vi "DAQAssist-2.vi"(0 "Calibration Array":dbl[](array[numeric]), 1 "number of samples":i32, 2 "rate":dbl, 3 "error in":errorcluster, 4 "stopped":bool) -> (5 "Dynamic Data Type":dynamicdata(waveform), 6 "error out":errorcluster)   [LabVIEW 2012]
uses:
  <vilib>/DAQmx/read.llb/DAQmx Read (Analog 1D Wfm NChan NSamp).vi
  <vilib>/DAQmx/create/channels.llb/DAQmx Create Channel (TEDS-AI-Voltage-Basic).vi
  <vilib>/DAQmx/create/channels.llb/DAQmx Create Channel (AI-Voltage-Basic).vi
  <vilib>/DAQmx/create/channels.llb/DAQmx Create Channel (TEDS-AI-Acceleration-Accelerometer).vi
  <vilib>/DAQmx/create/channels.llb/DAQmx Create Channel (AI-Acceleration-Accelerometer).vi
  <vilib>/DAQmx/configure/timing.llb/DAQmx Timing (Sample Clock).vi
  <vilib>/DAQmx/miscellaneous.llb/DAQmx Fill In Error Info.vi
  <resource>/objmgr/daqmx.rc
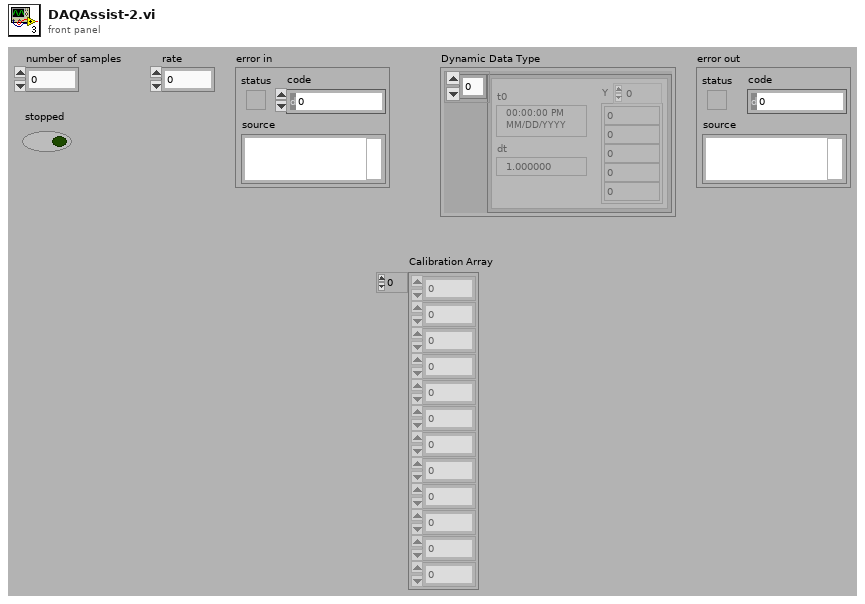
[diagram p1: front panel]
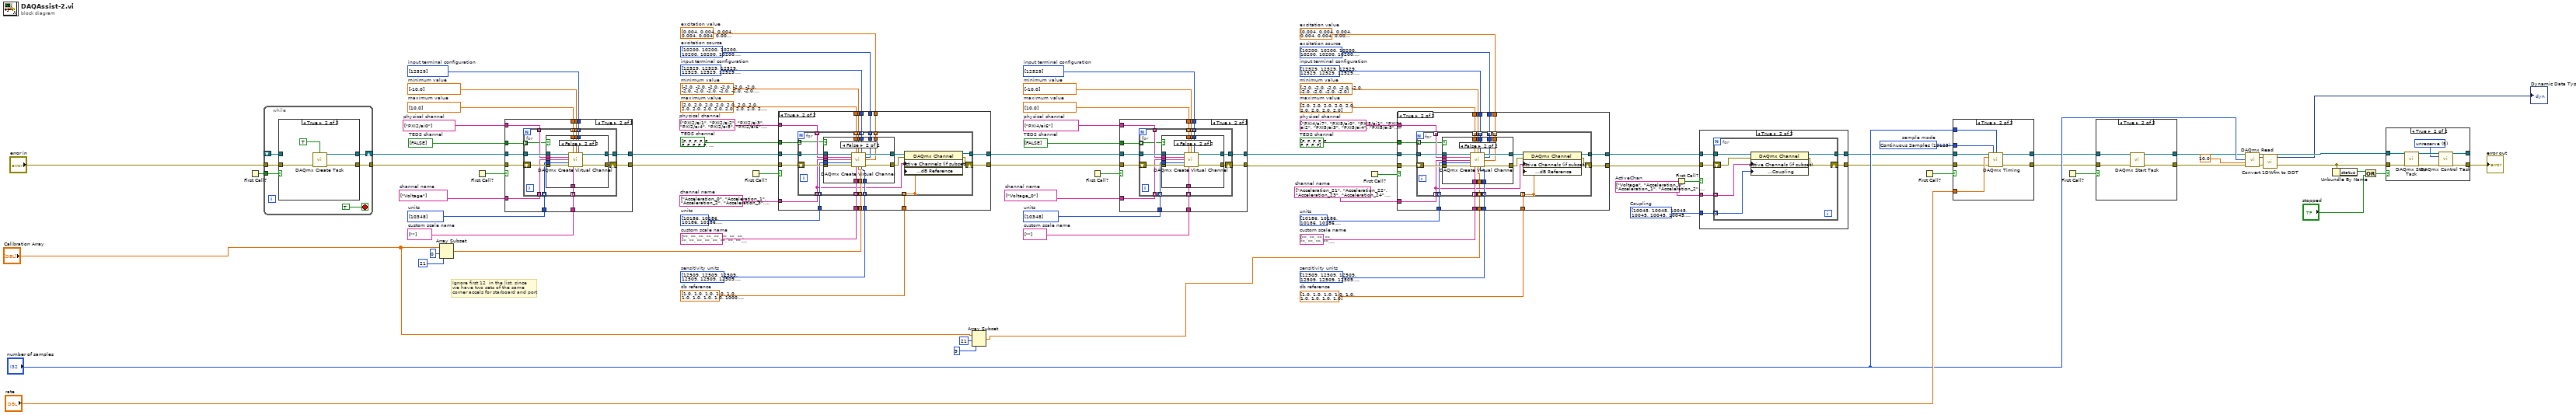
[diagram p0: block diagram]
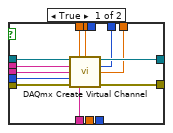
[diagram p3: hidden frame]
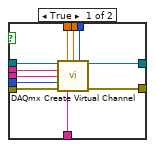
[diagram p5: hidden frame]
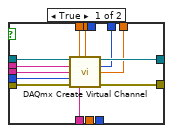
[diagram p11: hidden frame]
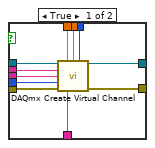
[diagram p13: hidden frame]
diagram:
  w9 = string[] ["Acceleration_21", "Acceleration_22", "Acceleration_23", "Acceleration_24", "Acceleration_25", "Acceleration_26", "Acceleration_27", "Acceleration_28", "Acceleration_29"]  # channel name
  w10 = string[] ["Voltage_0"]  # channel name
  w11 = string[] ["Acceleration_0", "Acceleration_1", "Acceleration_2", "Acceleration_3", "Acceleration_4", "Acceleration_5", "Acceleration_6", "Acceleration_7", "Acceleration_8", "Acceleration_9", "Acceleration_10", "Acceleration_11", "Acceleration_12", "Acceleration_13", "Acceleration_14", "Acceleration_15", "Acceleration_16", "Acceleration_17", "Acceleration_18", "Acceleration_19", "Acceleration_20"]  # channel name
  w12 = string[] ["PXI2/ai1", "PXI2/ai2", "PXI2/ai3", "PXI2/ai4", "PXI2/ai5", "PXI2/ai6", "PXI2/ai7", "PXI3/ai0", "PXI3/ai1", "PXI3/ai2", "PXI3/ai3", "PXI3/ai4", "PXI3/ai5", "PXI3/ai6", "PXI3/ai7", "PXI4/ai0", "PXI4/ai1", "PXI4/ai2", "PXI4/ai3", "PXI4/ai4", "PXI4/ai5"]  # physical channel
  w13 = string[] ["Voltage"]  # channel name
  w14 = string[] ["PXI2/ai0"]  # physical channel
  w15 = i32[] [10045, 10045, 10045, 10045, 10045, 10045, 10045, 10045, 10045, 10045, 10045, 10045, 10045, 10045, 10045, 10045, 10045, 10045, 10045, 10045, 10045, 10045, 10045, 10045, 10045, 10045, 10045, 10045, 10045, 10045, 10045, 10045] items=["AC"=10045, "DC"=10050, "GND"=10066]  # Coupling
  w16 = string[] ["Voltage", "Acceleration_0", "Acceleration_1", "Acceleration_2", "Acceleration_3", "Acceleration_4", "Acceleration_5", "Acceleration_6", "Acceleration_7", "Acceleration_8", "Acceleration_9", "Acceleration_10", "Acceleration_11", "Acceleration_12", "Acceleration_13", "Acceleration_14", "Acceleration_15", "Acceleration_16", "Acceleration_17", "Acceleration_18", "Acceleration_19", "Acceleration_20", "Voltage_0", "Acceleration_21", "Acceleration_22", "Acceleration_23", "Acceleration_24", "Acceleration_25", "Acceleration_26", "Acceleration_27", "Acceleration_28", "Acceleration_29"]  # ActiveChan
  w32 = dbl[] [1.0, 1.0, 1.0, 1.0, 1.0, 1.0, 1.0, 1.0, 1.0]  # db reference
  w31 = bool[] [FALSE, FALSE, FALSE, FALSE, FALSE, FALSE, FALSE, FALSE, FALSE]  # TEDS channel
  w30 = i32[] [12529, 12529, 12529, 12529, 12529, 12529, 12529, 12529, 12529] items=["default"=-1, "RSE"=10083, "NRSE"=10078, "Differential"=10106, "Pseudodifferential"=12529]  # input terminal configuration
  w28 = i32[] [10200, 10200, 10200, 10200, 10200, 10200, 10200, 10200, 10200] items=["Internal"=10200, "External"=10167, "None"=10230]  # excitation source
  w29 = i32[] [12509, 12509, 12509, 12509, 12509, 12509, 12509, 12509, 12509] items=["mVolts/g"=12509, "Volts/g"=12510]  # sensitivity units
  w27 = dbl[] [0.004, 0.004, 0.004, 0.004, 0.004, 0.004, 0.004, 0.004, 0.004]  # excitation value
  w26 = string[] ["", "", "", "", "", "", "", "", ""]  # custom scale name
  w25 = i32[] [10186, 10186, 10186, 10186, 10186, 10186, 10186, 10186, 10186] items=["g"=10186, "m/s^2"=12470, "From Custom Scale"=10065]  # units
  w24 = string[] ["PXI4/ai7", "PXI5/ai0", "PXI5/ai1", "PXI5/ai2", "PXI5/ai3", "PXI5/ai4", "PXI5/ai5", "PXI5/ai6", "PXI5/ai7"]  # physical channel
  w23 = dbl[] [2.0, 2.0, 2.0, 2.0, 2.0, 2.0, 2.0, 2.0, 2.0]  # maximum value
  w22 = dbl[] [-2.0, -2.0, -2.0, -2.0, -2.0, -2.0, -2.0, -2.0, -2.0]  # minimum value
  w42 = bool[] [FALSE]  # TEDS channel
  w41 = string[] [""]  # custom scale name
  w40 = i32[] [10348] items=["Volts"=10348, "From TEDS"=12516, "From Custom Scale"=10065]  # units
  w39 = string[] ["PXI4/ai6"]  # physical channel
  w38 = dbl[] [10.0]  # maximum value
  w37 = dbl[] [-10.0]  # minimum value
  w36 = i32[] [12529] items=["default"=-1, "RSE"=10083, "NRSE"=10078, "Differential"=10106, "Pseudodifferential"=12529]  # input terminal configuration
  w72 = 10123 items=["Finite Samples"=10178, "Continuous Samples"=10123, "Hardware Timed Single Point"=12522]  # sample mode
  w66 = dbl[] [1.0, 1.0, 1.0, 1.0, 1.0, 1.0, 1.0, 1.0, 1.0, 1000.0, 1000.0, 1000.0, 1000.0, 1000.0, 1000.0, 1000.0, 1000.0, 1000.0, 1000.0, 1000.0, 1.0]  # db reference
  w65 = bool[] [FALSE, FALSE, FALSE, FALSE, FALSE, FALSE, FALSE, FALSE, FALSE, FALSE, FALSE, FALSE, FALSE, FALSE, FALSE, FALSE, FALSE, FALSE, FALSE, FALSE, FALSE]  # TEDS channel
  w64 = i32[] [12529, 12529, 12529, 12529, 12529, 12529, 12529, 12529, 12529, 12529, 12529, 12529, 12529, 12529, 12529, 12529, 12529, 12529, 12529, 12529, 12529] items=["default"=-1, "RSE"=10083, "NRSE"=10078, "Differential"=10106, "Pseudodifferential"=12529]  # input terminal configuration
  w62 = i32[] [10200, 10200, 10200, 10200, 10200, 10200, 10200, 10200, 10200, 10200, 10200, 10200, 10200, 10200, 10200, 10200, 10200, 10200, 10200, 10200, 10200] items=["Internal"=10200, "External"=10167, "None"=10230]  # excitation source
  w63 = i32[] [12509, 12509, 12509, 12509, 12509, 12509, 12509, 12509, 12509, 12509, 12509, 12509, 12509, 12509, 12509, 12509, 12509, 12509, 12509, 12509, 12509] items=["mVolts/g"=12509, "Volts/g"=12510]  # sensitivity units
  w61 = dbl[] [0.004, 0.004, 0.004, 0.004, 0.004, 0.004, 0.004, 0.004, 0.004, 0.004, 0.004, 0.004, 0.004, 0.004, 0.004, 0.004, 0.004, 0.004, 0.004, 0.004, 0.004]  # excitation value
  w60 = string[] ["", "", "", "", "", "", "", "", "", "", "", "", "", "", "", "", "", "", "", "", ""]  # custom scale name
  w59 = i32[] [10186, 10186, 10186, 10186, 10186, 10186, 10186, 10186, 10186, 10186, 10186, 10186, 10186, 10186, 10186, 10186, 10186, 10186, 10186, 10186, 10186] items=["g"=10186, "m/s^2"=12470, "From Custom Scale"=10065]  # units
  w58 = dbl[] [2.0, 2.0, 2.0, 2.0, 2.0, 2.0, 2.0, 2.0, 2.0, 2.0, 2.0, 2.0, 2.0, 2.0, 2.0, 2.0, 2.0, 2.0, 2.0, 2.0, 2.0]  # maximum value
  w57 = dbl[] [-2.0, -2.0, -2.0, -2.0, -2.0, -2.0, -2.0, -2.0, -2.0, -2.0, -2.0, -2.0, -2.0, -2.0, -2.0, -2.0, -2.0, -2.0, -2.0, -2.0, -2.0]  # minimum value
  w54 = bool[] [FALSE]  # TEDS channel
  w53 = string[] [""]  # custom scale name
  w52 = i32[] [10348] items=["Volts"=10348, "From TEDS"=12516, "From Custom Scale"=10065]  # units
  w51 = dbl[] [10.0]  # maximum value
  w50 = dbl[] [-10.0]  # minimum value
  w49 = i32[] [12529] items=["default"=-1, "RSE"=10083, "NRSE"=10078, "Differential"=10106, "Pseudodifferential"=12529]  # input terminal configuration
  # "Ignore first 12  in the list, since \nwe have two sets of the same \ncorner accels for starboard and port"
  n1 = First Call?() -> (First Call?: T/F=w43:bool)
  n2 = while {
    shift-right: [w91] -> w47
    shift-left: _ -> [w90]
    tunnel: w43 -> [w92]
    tunnel: [w89] -> w44
    tunnel: "error in" -> [w88]
    stop <- TRUE stop-if-true
    n3 = case shown="True" w92 {
      tunnel: [w94 w98] -> w91
      tunnel: w90 -> [w94 _]
      tunnel: [w93 w97] -> w89
      tunnel: w88 -> [w93 w95]
      frame False {
      }
      frame True {
        n4 = call <vilib>:"DAQmx Create Task.vi"("auto cleanup"=TRUE, "error in"=w95) -> ("task out"=w98:refnum<k21>, "error out"=w97:errorcluster)  [unwired: 12 in]
      }
    }
  }
  n5 = Array Subset(array="Calibration Array", index=0, length=21) -> (w6:dbl[])
  n6 = First Call?() -> (First Call?: T/F=w46:bool)
  n7 = case shown="True" w46 {
    tunnel: [w100 w110] -> w56
    tunnel: w47 -> [w100 w112]
    tunnel: [w99 w109] -> w48
    tunnel: w44 -> [w99 w111]
    tunnel: w49 -> [_ w108]
    tunnel: w50 -> [_ w107]
    tunnel: w51 -> [_ w106]
    tunnel: w14 -> [_ w105]
    tunnel: w13 -> [_ w104]
    tunnel: w52 -> [_ w103]
    tunnel: w53 -> [_ w102]
    tunnel: w54 -> [_ w101]
    frame False {
    }
    frame True {
      n8 = for {
        tunnel: w112 -> [w124]
        tunnel: [w122] -> w110
        tunnel: w108 -> [w120] mode=indexing
        tunnel: w107 -> [w119] mode=indexing
        tunnel: w106 -> [w118] mode=indexing
        tunnel: w105 -> [w117] mode=indexing
        tunnel: w104 -> [w116] mode=indexing
        tunnel: w103 -> [w115] mode=indexing
        tunnel: w102 -> [w114] mode=indexing
        shift-right: [w121] -> w109
        shift-left: w111 -> [w123]
        tunnel: w101 -> [w113] mode=indexing
        n9 = case shown="False" w113 {
          tunnel: w124 -> [w135 w146]
          tunnel: w123 -> [w134 w145]
          tunnel: [w133 w144] -> w122
          tunnel: [w132 w143] -> w121
          tunnel: w120 -> [w131 w142]
          tunnel: w119 -> [w130 w141]
          tunnel: w118 -> [w129 w140]
          tunnel: w117 -> [w128 w139]
          tunnel: w116 -> [w127 w138]
          tunnel: w115 -> [w126 w137]
          tunnel: w114 -> [w125 w136]
          frame True {
            n10 = call-poly <vilib>:"DAQmx Create Virtual Channel.vi"("task in"=w135, "maximum value"=w129, "minimum value"=w130, "input terminal configuration"=w131, "physical channels"=w128, "name to assign"=w127, "units"=w126, "error in"=w134, "custom scale name"=w125) -> ("task out"=w133:refnum<k21>, "error out"=w132:errorcluster)  [unwired: 5 in]
          }
          frame False {
            n11 = call-poly <vilib>:"DAQmx Create Virtual Channel.vi"("task in"=w146, "maximum value"=w140, "minimum value"=w141, "input terminal configuration"=w142, "physical channels"=w139, "name to assign"=w138, "units"=w137, "error in"=w145, "custom scale name"=w136) -> ("task out"=w144:refnum<k21>, "error out"=w143:errorcluster)  [unwired: 5 in]
          }
        }
      }
    }
  }
  n12 = First Call?() -> (First Call?: T/F=w55:bool)
  n13 = case shown="True" w55 {
    tunnel: [w148 w163] -> w34
    tunnel: w56 -> [w148 w165]
    tunnel: [w147 w162] -> w33
    tunnel: w48 -> [w147 w164]
    tunnel: w57 -> [_ w161]
    tunnel: w58 -> [_ w160]
    tunnel: w12 -> [_ w159]
    tunnel: w11 -> [_ w158]
    tunnel: w59 -> [_ w157]
    tunnel: w60 -> [_ w156]
    tunnel: w61 -> [_ w155]
    tunnel: w62 -> [_ w154]
    tunnel: w6 -> [_ w153]
    tunnel: w63 -> [_ w152]
    tunnel: w64 -> [_ w151]
    tunnel: w65 -> [_ w150]
    tunnel: w66 -> [_ w149]
    frame False {
    }
    frame True {
      n14 = for {
        tunnel: w165 -> [w184]
        tunnel: [w170] -> w163
        tunnel: w161 -> [w182] mode=indexing
        tunnel: w160 -> [w181] mode=indexing
        tunnel: w159 -> [w180] mode=indexing
        tunnel: w158 -> [w166] mode=indexing
        tunnel: w157 -> [w179] mode=indexing
        tunnel: w156 -> [w178] mode=indexing
        shift-right: [w169] -> w162
        shift-left: w164 -> [w183]
        tunnel: w155 -> [w177] mode=indexing
        tunnel: w154 -> [w176] mode=indexing
        tunnel: w153 -> [w175] mode=indexing
        tunnel: w152 -> [w174] mode=indexing
        tunnel: w151 -> [w173] mode=indexing
        tunnel: w150 -> [w172] mode=indexing
        tunnel: [w167] -> _ mode=indexing
        tunnel: w149 -> [w167] mode=indexing
        n15 = case shown="False" w172 {
          tunnel: w184 -> [w196 w211]
          tunnel: w183 -> [w195 w210]
          tunnel: [w194 w209] -> w171
          tunnel: [w193 w208] -> w168
          tunnel: w182 -> [w192 w207]
          tunnel: w181 -> [w191 w206]
          tunnel: w180 -> [w190 w205]
          tunnel: w166 -> [w189 w204]
          tunnel: w179 -> [w188 w203]
          tunnel: w178 -> [w187 w202]
          tunnel: w177 -> [w186 w201]
          tunnel: w176 -> [w185 w200]
          tunnel: w175 -> [_ w199]
          tunnel: w174 -> [_ w198]
          tunnel: w173 -> [_ w197]
          frame True {
            n16 = call-poly <vilib>:"DAQmx Create Virtual Channel.vi"("task in"=w196, "maximum value"=w191, "minimum value"=w192, "physical channels"=w190, "current excitation source"=w185, "name to assign"=w189, "current excitation value"=w186, "units"=w188, "error in"=w195, "custom scale name"=w187) -> ("task out"=w194:refnum<k21>, "error out"=w193:errorcluster)  [unwired: 4 in]
          }
          frame False {
            n17 = call-poly <vilib>:"DAQmx Create Virtual Channel.vi"("task in"=w211, "maximum value"=w206, "minimum value"=w207, "input terminal configuration"=w197, "physical channels"=w205, "current excitation source"=w200, "name to assign"=w204, "current excitation value"=w201, "units"=w203, "error in"=w210, "custom scale name"=w202, "sensitivity"=w199, "sensitivity units"=w198) -> ("task out"=w209:refnum<k21>, "error out"=w208:errorcluster)  [unwired: 1 in]
          }
        }
        n18 = property class="DAQmx Channel"(reference=w171, error in=w168, "Active Channels (if subset)"=w166, "Analog Input:Acceleration:dB Reference"=w167) -> (reference out=w170:refnum<k21>, error out=w169:errorcluster)
      }
    }
  }
  n19 = Array Subset(array="Calibration Array", index=21, length=9) -> (w2:dbl[])
  n20 = First Call?() -> (First Call?: T/F=w35:bool)
  n21 = case shown="True" w35 {
    tunnel: [w213 w223] -> w20
    tunnel: w34 -> [w213 w225]
    tunnel: [w212 w222] -> w19
    tunnel: w33 -> [w212 w224]
    tunnel: w36 -> [_ w221]
    tunnel: w37 -> [_ w220]
    tunnel: w38 -> [_ w219]
    tunnel: w39 -> [_ w218]
    tunnel: w10 -> [_ w217]
    tunnel: w40 -> [_ w216]
    tunnel: w41 -> [_ w215]
    tunnel: w42 -> [_ w214]
    frame False {
    }
    frame True {
      n22 = for {
        tunnel: w225 -> [w237]
        tunnel: [w235] -> w223
        tunnel: w221 -> [w233] mode=indexing
        tunnel: w220 -> [w232] mode=indexing
        tunnel: w219 -> [w231] mode=indexing
        tunnel: w218 -> [w230] mode=indexing
        tunnel: w217 -> [w229] mode=indexing
        tunnel: w216 -> [w228] mode=indexing
        tunnel: w215 -> [w227] mode=indexing
        shift-right: [w234] -> w222
        shift-left: w224 -> [w236]
        tunnel: w214 -> [w226] mode=indexing
        n23 = case shown="False" w226 {
          tunnel: w237 -> [w248 w259]
          tunnel: w236 -> [w247 w258]
          tunnel: [w246 w257] -> w235
          tunnel: [w245 w256] -> w234
          tunnel: w233 -> [w244 w255]
          tunnel: w232 -> [w243 w254]
          tunnel: w231 -> [w242 w253]
          tunnel: w230 -> [w241 w252]
          tunnel: w229 -> [w240 w251]
          tunnel: w228 -> [w239 w250]
          tunnel: w227 -> [w238 w249]
          frame True {
            n24 = call-poly <vilib>:"DAQmx Create Virtual Channel.vi"("task in"=w248, "maximum value"=w242, "minimum value"=w243, "input terminal configuration"=w244, "physical channels"=w241, "name to assign"=w240, "units"=w239, "error in"=w247, "custom scale name"=w238) -> ("task out"=w246:refnum<k21>, "error out"=w245:errorcluster)  [unwired: 5 in]
          }
          frame False {
            n25 = call-poly <vilib>:"DAQmx Create Virtual Channel.vi"("task in"=w259, "maximum value"=w253, "minimum value"=w254, "input terminal configuration"=w255, "physical channels"=w252, "name to assign"=w251, "units"=w250, "error in"=w258, "custom scale name"=w249) -> ("task out"=w257:refnum<k21>, "error out"=w256:errorcluster)  [unwired: 5 in]
          }
        }
      }
    }
  }
  n26 = First Call?() -> (First Call?: T/F=w21:bool)
  n27 = case shown="True" w21 {
    tunnel: [w261 w276] -> w18
    tunnel: w20 -> [w261 w278]
    tunnel: [w260 w275] -> w17
    tunnel: w19 -> [w260 w277]
    tunnel: w22 -> [_ w274]
    tunnel: w23 -> [_ w273]
    tunnel: w24 -> [_ w272]
    tunnel: w9 -> [_ w271]
    tunnel: w25 -> [_ w270]
    tunnel: w26 -> [_ w269]
    tunnel: w27 -> [_ w268]
    tunnel: w28 -> [_ w267]
    tunnel: w29 -> [_ w266]
    tunnel: w30 -> [_ w265]
    tunnel: w31 -> [_ w264]
    tunnel: w32 -> [_ w263]
    tunnel: w2 -> [_ w262]
    frame False {
    }
    frame True {
      n28 = for {
        tunnel: w278 -> [w297]
        tunnel: [w284] -> w276
        tunnel: w274 -> [w295] mode=indexing
        tunnel: w273 -> [w294] mode=indexing
        tunnel: w272 -> [w293] mode=indexing
        tunnel: w271 -> [w280] mode=indexing
        tunnel: w270 -> [w292] mode=indexing
        tunnel: w269 -> [w291] mode=indexing
        shift-right: [w283] -> w275
        shift-left: w277 -> [w296]
        tunnel: w268 -> [w290] mode=indexing
        tunnel: w267 -> [w289] mode=indexing
        tunnel: w266 -> [w288] mode=indexing
        tunnel: w265 -> [w287] mode=indexing
        tunnel: w264 -> [w286] mode=indexing
        tunnel: [w281] -> _ mode=indexing
        tunnel: w263 -> [w281] mode=indexing
        tunnel: w262 -> [w279] mode=indexing
        n29 = case shown="False" w286 {
          tunnel: w297 -> [w309 w324]
          tunnel: w296 -> [w308 w323]
          tunnel: [w307 w322] -> w285
          tunnel: [w306 w321] -> w282
          tunnel: w295 -> [w305 w320]
          tunnel: w294 -> [w304 w319]
          tunnel: w293 -> [w303 w318]
          tunnel: w280 -> [w302 w317]
          tunnel: w292 -> [w301 w316]
          tunnel: w291 -> [w300 w315]
          tunnel: w290 -> [w299 w314]
          tunnel: w289 -> [w298 w313]
          tunnel: w288 -> [_ w312]
          tunnel: w287 -> [_ w311]
          tunnel: w279 -> [_ w310]
          frame True {
            n30 = call-poly <vilib>:"DAQmx Create Virtual Channel.vi"("task in"=w309, "maximum value"=w304, "minimum value"=w305, "physical channels"=w303, "current excitation source"=w298, "name to assign"=w302, "current excitation value"=w299, "units"=w301, "error in"=w308, "custom scale name"=w300) -> ("task out"=w307:refnum<k21>, "error out"=w306:errorcluster)  [unwired: 4 in]
          }
          frame False {
            n31 = call-poly <vilib>:"DAQmx Create Virtual Channel.vi"("task in"=w324, "maximum value"=w319, "minimum value"=w320, "input terminal configuration"=w311, "physical channels"=w318, "current excitation source"=w313, "name to assign"=w317, "current excitation value"=w314, "units"=w316, "error in"=w323, "custom scale name"=w315, "sensitivity"=w310, "sensitivity units"=w312) -> ("task out"=w322:refnum<k21>, "error out"=w321:errorcluster)  [unwired: 1 in]
          }
        }
        n32 = property class="DAQmx Channel"(reference=w285, error in=w282, "Active Channels (if subset)"=w280, "Analog Input:Acceleration:dB Reference"=w281) -> (reference out=w284:refnum<k21>, error out=w283:errorcluster)
      }
    }
  }
  n33 = First Call?() -> (First Call?: T/F=w68:bool)
  n34 = case shown="True" w68 {
    tunnel: w18 -> [w326 w332]
    tunnel: w17 -> [w325 w331]
    tunnel: [w326 w330] -> w70
    tunnel: [w325 w329] -> w67
    tunnel: w16 -> [_ w328]
    tunnel: w15 -> [_ w327]
    frame False {
    }
    frame True {
      n35 = for {
        tunnel: w332 -> [w338]
        tunnel: [w336] -> w330
        tunnel: w328 -> [w334] mode=indexing
        shift-right: [w335] -> w329
        shift-left: w331 -> [w337]
        tunnel: w327 -> [w333] mode=indexing
        n36 = property class="DAQmx Channel"(reference=w338, error in=w337, "Active Channels (if subset)"=w334, "Analog Input:General Properties:Input Configuration:Coupling"=w333) -> (reference out=w336:refnum<k21>, error out=w335:errorcluster)
      }
    }
  }
  n37 = First Call?() -> (First Call?: T/F=w69:bool)
  n38 = case shown="True" w69 {
    tunnel: [w340 w342] -> w74
    tunnel: w70 -> [w340 w345]
    tunnel: [w339 w341] -> w71
    tunnel: w67 -> [w339 w343]
    tunnel: "number of samples" -> [_ w347]
    tunnel: w72 -> [_ w346]
    tunnel: "rate" -> [_ w344]
    frame False {
    }
    frame True {
      n39 = call-poly <vilib>:"DAQmx Timing.vi"("task/channels in"=w345, "sample mode"=w346, "samples per channel"=w347, "rate"=w344, "error in"=w343) -> ("task out"=w342:refnum<k21>, "error out"=w341:errorcluster)  [unwired: 9 in]
    }
  }
  n40 = First Call?() -> (First Call?: T/F=w73:bool)
  n41 = case shown="True" w73 {
    tunnel: [w349 w352] -> w77
    tunnel: w74 -> [w349 w353]
    tunnel: [w348 w350] -> w75
    tunnel: w71 -> [w348 w351]
    frame False {
    }
    frame True {
      n42 = call <vilib>:"DAQmx Start Task.vi"("task/channels in"=w353, "error in"=w351) -> ("task out"=w352:refnum<k21>, "error out"=w350:errorcluster)  [unwired: 12 in]
    }
  }
  n43 = call-poly <vilib>:"DAQmx Read.vi"("task/channels in"=w77, "number of samples per channel"="number of samples", "timeout"=10.0, "error in"=w75) -> ("task out"=w81:refnum<k21>, "data"=w79:waveform(dbl)[], "error out"=w76:errorcluster)  [unwired: 9 in]
  n44 = call <vilib>:"Convert 1DWfm to DDT.vi"("Array of Waveforms"=w79) -> ("Dynamic Data Type"=→"Dynamic Data Type":dynamicdata)  [unwired: 3 in]
  n45 = Unbundle By Name(w76) -> ("status"=w83:bool)
  n46 = Or(x=w83, y="stopped") -> (x .or. y?=w84:bool)
  n47 = case shown="True" w84 {
    tunnel: [w355 w356] -> _
    tunnel: w81 -> [w355 w362]
    tunnel: [w354 w359] -> w82
    tunnel: w76 -> [w354 w361]
    frame False {
    }
    frame True {
      w357 = 5 items=["verify"=2, "reserve"=4, "commit"=3, "unreserve"=5, "abort"=6] ("action")
      n48 = call <vilib>:"DAQmx Stop Task.vi"("task/channels in"=w362, "error in"=w361) -> ("task out"=w358:refnum<k21>, "error out"=w360:errorcluster)  [unwired: 12 in]
      n49 = call <vilib>:"DAQmx Control Task.vi"("task/channels in"=w358, "action"=w357, "error in"=w360) -> ("task out"=w356:refnum<k21>, "error out"=w359:errorcluster)  [unwired: 11 in]
    }
  }
  "error out" <- w82
